vi "4) (a) Using Sub VI (Temperature Conversion).vi"() -> ()   [LabVIEW 2018]
panel:
  in  "Switch":bool
  in  "Temperature (F)":dbl(slide) scale=0.0..100.0
  out "Temperature (C)":dbl(slide) scale=0.0..100.0
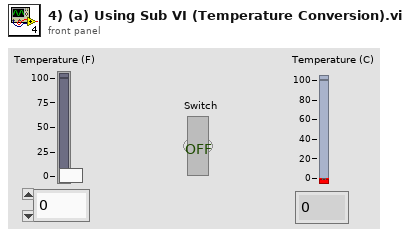
[diagram p1: front panel]
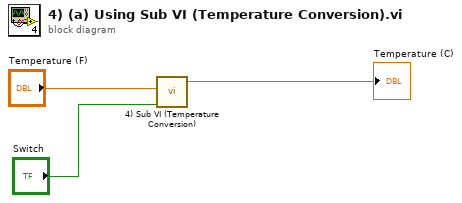
[diagram p0: block diagram]
diagram:
  n1 = call "4) Sub VI (Temperature Conversion).vi"("Boolean"="Switch", "Temperature (F)"="Temperature (F)") -> ("Numeric"=→"Temperature (C)":dbl)  [unwired: 9 in]
